vi "Amium Kommandos vorhanden - Prüfen.vi"(10 "Vorhanden??":string[](array[string]), 11 "Kommandos":string[](array[string])) -> (3 "Kommandos":string[](array[string]))   [LabVIEW 2020, in "Amium PNS.lvlib" / "AK Kommunikation.lvlib"]
uses:
  AK Kommunikation.lvlib
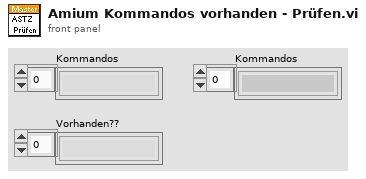
[diagram p1: front panel]
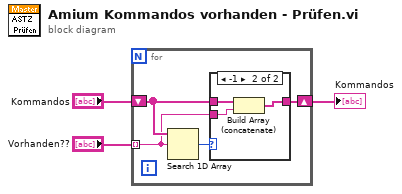
[diagram p0: block diagram]
diagram:
  n1 = for {
    tunnel: "Vorhanden??" -> [w5] mode=indexing
    shift-right: [w4] -> w2
    shift-left: "Kommandos" -> [w6]
    n2 = Search 1D Array(1D array=w6, element=w5) -> (index of element=w7:i32)  [unwired: 1 in]
    n3 = case shown="-1" w7 {
      tunnel: w6 -> [w8 w11]
      tunnel: w5 -> [_ w10]
      tunnel: [w8 w9] -> w4
      frame 0, Default {
      }
      frame -1 {
        n4 = Build Array (concatenate)(w11, w10) -> (w9:string[])
      }
    }
  }
  "Kommandos" <- w2
